vi "String_ErrorMessageContainsString.vi"() -> ()   [LabVIEW 2017, in "AssertionTest.lvlib" / "AssertIsBoolean.lvlib"]
uses:
  AssertIsBoolean.lvlib
  Assertion/Assertion.lvlib
panel:
  out "error out":errorcluster
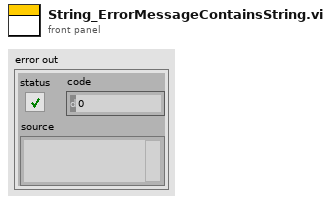
[diagram p1: front panel]
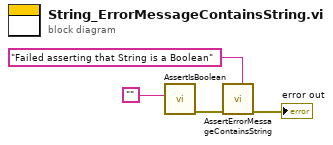
[diagram p0: block diagram]
diagram:
  n1 = call "AssertIsBoolean.vi"("Actual"="") -> ("error out"=w3:errorcluster)  [unwired: 10 in]
  n2 = call "AssertErrorMessageContainsString.vi"("Expected"="Failed asserting that String is a Boolean", "error in (no error)"=w3) -> ("error out"=→"error out":errorcluster)  [unwired: 9 in]
